vi "ReadOVABinFile.vi"(0 "Measurement Data File Path":path, 1 "Target Matrix":u8(ring) items=["A", "B", "C"], 2 "Allow MessageBoxes?":bool=TRUE, 5 "error in (no error)":errorcluster) -> (19 "error out":errorcluster)   [LabVIEW 2012]
doc: "Reads measurement data stored in a binary data file specified to the enumerated measClass object. Subsequently, it sets up the time domain window, either to a default region, or to the saved window region for the enumerated measurement, depending on whether any preexisting window was flagged to be retained."
uses:
  bin/OVA32.dll
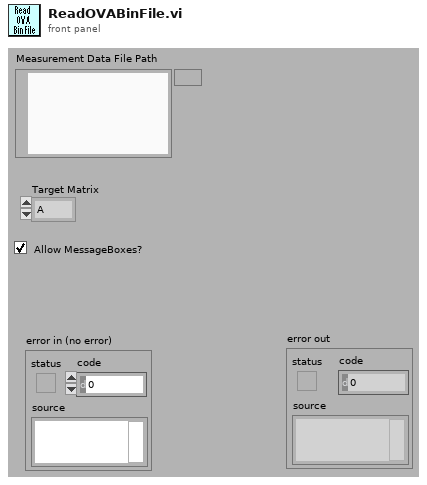
[diagram p1: front panel]
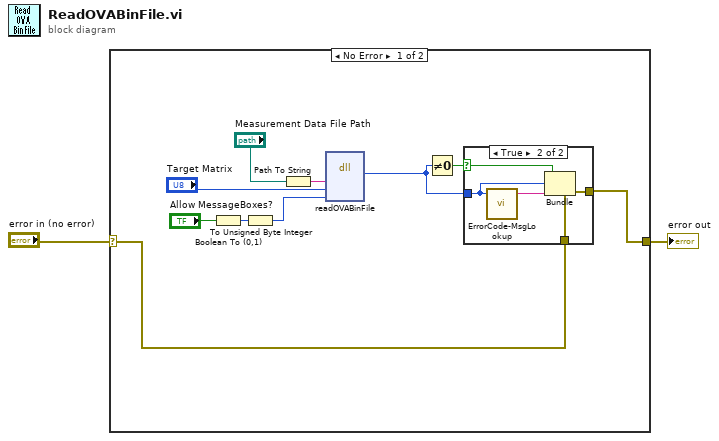
[diagram p0: block diagram]
diagram:
  n1 = case shown="No Error" "error in (no error)" {
    selector: "error in (no error)" -> [w5 w19]
    tunnel: [w4 w19] -> w1
    frame No Error {
      n2 = Boolean To (0,1)(Boolean="Allow MessageBoxes?") -> (0, 1=w7:i16)
      n3 = To Unsigned Byte Integer(number=w7) -> (unsigned 8bit integer=w6:u8)
      n4 = Path To String(path="Measurement Data File Path") -> (string=w11:string)
      n5 = dll-call lib="C:/_src/OVA5000_DSP_falcon/Software/LabVIEW/OVA/SDK/OVA_5000_SDK_v5.14.3/bin/OVA32.dll" fn="readOVABinFile" label="readOVABinFile()"("OVABinFileName"=w11, "measSelection"="Target Matrix", "dialogAllowed"=w6) -> (w3:i32)  [unwired: 6 in, 2 out]
      n6 = Not Equal To 0?(x=w3) -> (x != 0?=w12:bool)
      n7 = case shown="True" w12 {
        selector: w12 -> [_ w15]
        tunnel: w3 -> [_ w16]
        tunnel: w5 -> [w13 w18]
        tunnel: [w13 w14] -> w4
        frame False {
        }
        frame True {
          n8 = call "ErrorCode-MsgLookup.vi"("DLL Return Code"=w16) -> ("Error String"=w17:string)  [unwired: 2 in, 2 out]
          n9 = Bundle(cluster=w18, "status"=w15, "code"=w16, "source"=w17) -> (w14:errorcluster)
        }
      }
    }
    frame Error {
    }
  }
  "error out" <- w1
